vi "Execute Command (Device).vi"(0 "SLSC Interface in":refnum<class "SLSC Interface.lvclass">, 5 "devices":refnum<k21>="$DefaultDevices", 7 "command":refnum<k21>, 11 "error in (no error)":errorcluster, 12 "timeout (10 sec)":dbl=10.0) -> (4 "SLSC Interface out":refnum<class "SLSC Interface.lvclass">, 15 "error out":errorcluster)   [LabVIEW 2015, in "SLSC Interface.lvclass"]
uses:
  SLSC Interface.lvclass
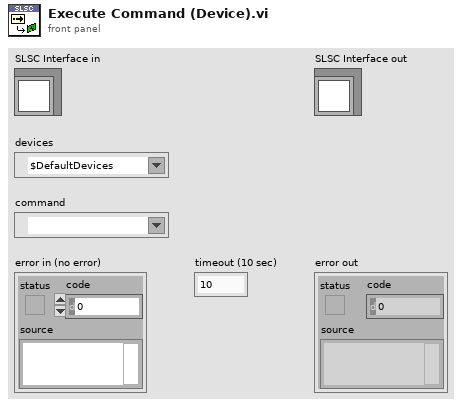
[diagram p1: front panel]
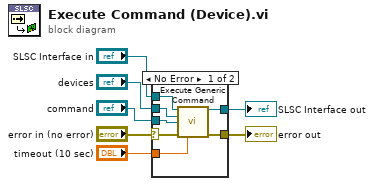
[diagram p0: block diagram]
diagram:
  n1 = case shown="No Error" "error in (no error)" {
    selector: "error in (no error)" -> [w10 w16]
    tunnel: [w9 w16] -> w6
    tunnel: [w13 w15] -> w4
    tunnel: "SLSC Interface in" -> [w14 w15]
    tunnel: "devices" -> [w12 _]
    tunnel: "command" -> [w11 _]
    tunnel: "timeout (10 sec)" -> [w8 _]
    frame No Error {
      n2 = call-dynamic "Execute Generic Command.vi"("SLSC Interface in"=w14, "resources"=w12, "command"=w11, "error in (no error)"=w10, "timeout (10 sec)"=w8) -> ("SLSC Interface out"=w13:refnum<class "SLSC Interface.lvclass">, "error out"=w9:errorcluster)  [unwired: 9 in]
    }
    frame Error {
    }
  }
  "error out" <- w6
  "SLSC Interface out" <- w4
